vi "Detector Send New Image Message.vi"(8 "error in (no error)":errorcluster, 11 "New Images":T2[](array[typedef]) {"Detector #" items=["None", "YJ", "HK"]}) -> (0 "error out":errorcluster, 3 "Image Messages":T1[](array[typedef]) {"Detector #" items=["None", "YJ", "HK"]})   [LabVIEW 2024]
uses:
  Detector Image typedef cluster.ctl
  Subsystems/SS cluster New Image Data.ctl
  Detector Class.lvclass
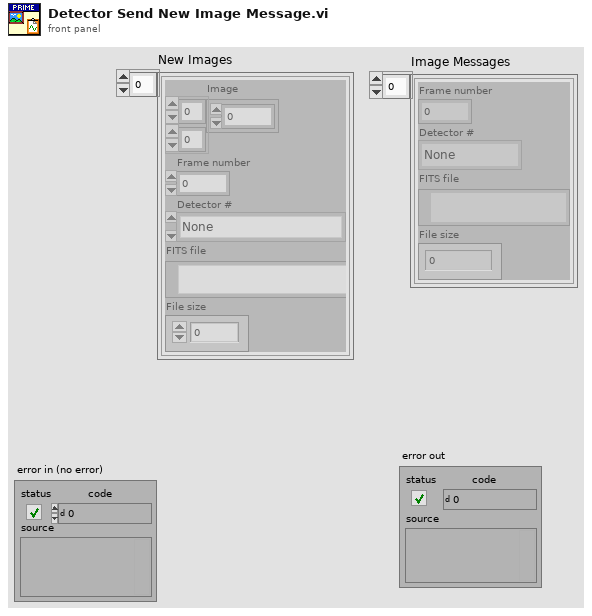
[diagram p1: front panel]
types:
  T1 = typedef "SS cluster New Image Data.ctl" = cluster{"Frame number":i32, "Detector #":u16, "FITS file":path, "File size":i64}
  T2 = typedef "Detector Class.lvclass/Detector Image typedef cluster.ctl" = cluster{"Image":sgl[][], "Frame number":i32, "Detector #":u16, "FITS file":path, "File size":i64}
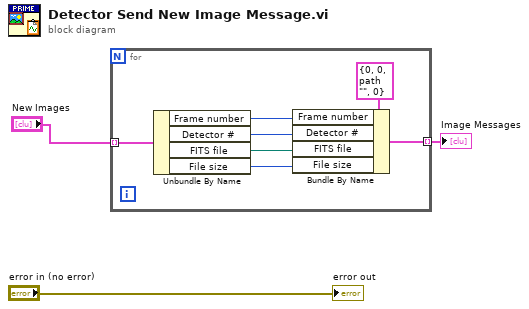
[diagram p0: block diagram]
diagram:
  n1 = for {
    tunnel: "New Images" -> [w5] mode=indexing
    tunnel: [w4] -> w1 mode=indexing
    n2 = Unbundle By Name(w5) -> ("Frame number"=w9:i32, "Detector #"=w8:u16, "FITS file"=w7:path, "File size"=w6:i64)
    n3 = Bundle By Name(cluster=T1 {"Frame number"=0, "Detector #"=0, "FITS file"=path "", "File size"=0} ("New Image"), "Frame number"=w9, "Detector #"=w8, "FITS file"=w7, "File size"=w6) -> (w4:T1)
  }
  "Image Messages" <- w1
  "error out" <- "error in (no error)"
